vi "Response Type.vi"(8 "error in (no error)":errorcluster, 11 "net-http-client in":refnum<class "net-http-client.lvclass">) -> (0 "error out":errorcluster, 2 "response type":refnum<class "response.lvclass">, 3 "net-http-client out":refnum<class "net-http-client.lvclass">)   [LabVIEW 2020, in "net-http-client.lvclass"]
uses:
  net-http-client.lvclass
  classes/response/response.lvclass
  net-response/net-response.lvclass
  C:/Viviota/Projects/R&D/LabVIEW_HTTP_REST_Client/source/classes/response/response.lvclass
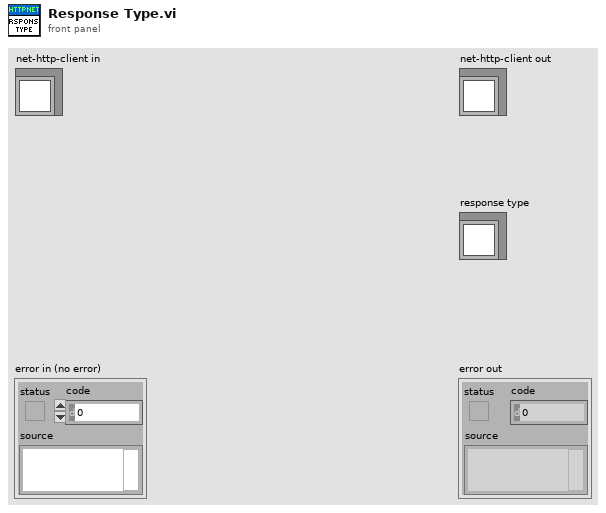
[diagram p1: front panel]
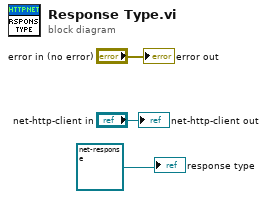
[diagram p0: block diagram]
diagram:
  "error out" <- "error in (no error)"
  "response type" <- refnum<class "net-response.lvclass"> refnum ("net-response.lvclass")
  "net-http-client out" <- "net-http-client in"
